vi "VI_Heat_Tape_Final_single_unit.vi"() -> ()   [LabVIEW 2019]
uses:
  <vilib>/NI/Modbus Library/API/Wrapper/Create Serial Master.vi
  <vilib>/NI/Modbus Library/API/Master/Modbus Master.lvclass
  <vilib>/NI/Modbus Library/API/Wrapper/API Main.lvlib
panel:
  out "Value 4":sgl
  out "Connection Status":bool
  in  "unit ID (Defaut: 1)":u8=1
  in  "number of inputs (Defaut: 60)":u16
  in  "starting address (Default: 1)":u16
  in  "Flow Control (Default: None)":u16(ring) items=["None", "XON/XOFF", "RTS/CTS", "XON/XOFF & RTS/CTS", "DTR/DSR", "XON/XOFF & DTR/DSR"]
  in  "Serial Type (Default: RTU)":enum16{"RTU", "ASCII"}(ring)
  in  "Parity (Default: None)":u16(ring)=2 items=["None", "Odd", "Even", "Mark", "Space"]
  in  "Baud Rate (Default: 115400)":u32=9600
  in  "COM Port (Default: COM7)":refnum<visa-resource-name>
  in  "Set Value":string
  out "?":cluster{dbl, dbl}(graph)
  in  "Hysterisis Value":string
  in  "?":bool
  out "Current Temperature (ºF)":string
  in  "error check":errorcluster
  # "SpinQuest Heat Tape Temperature Monitoring System"
  # "PXF4 Settings"
  # "RS-485 Connection"
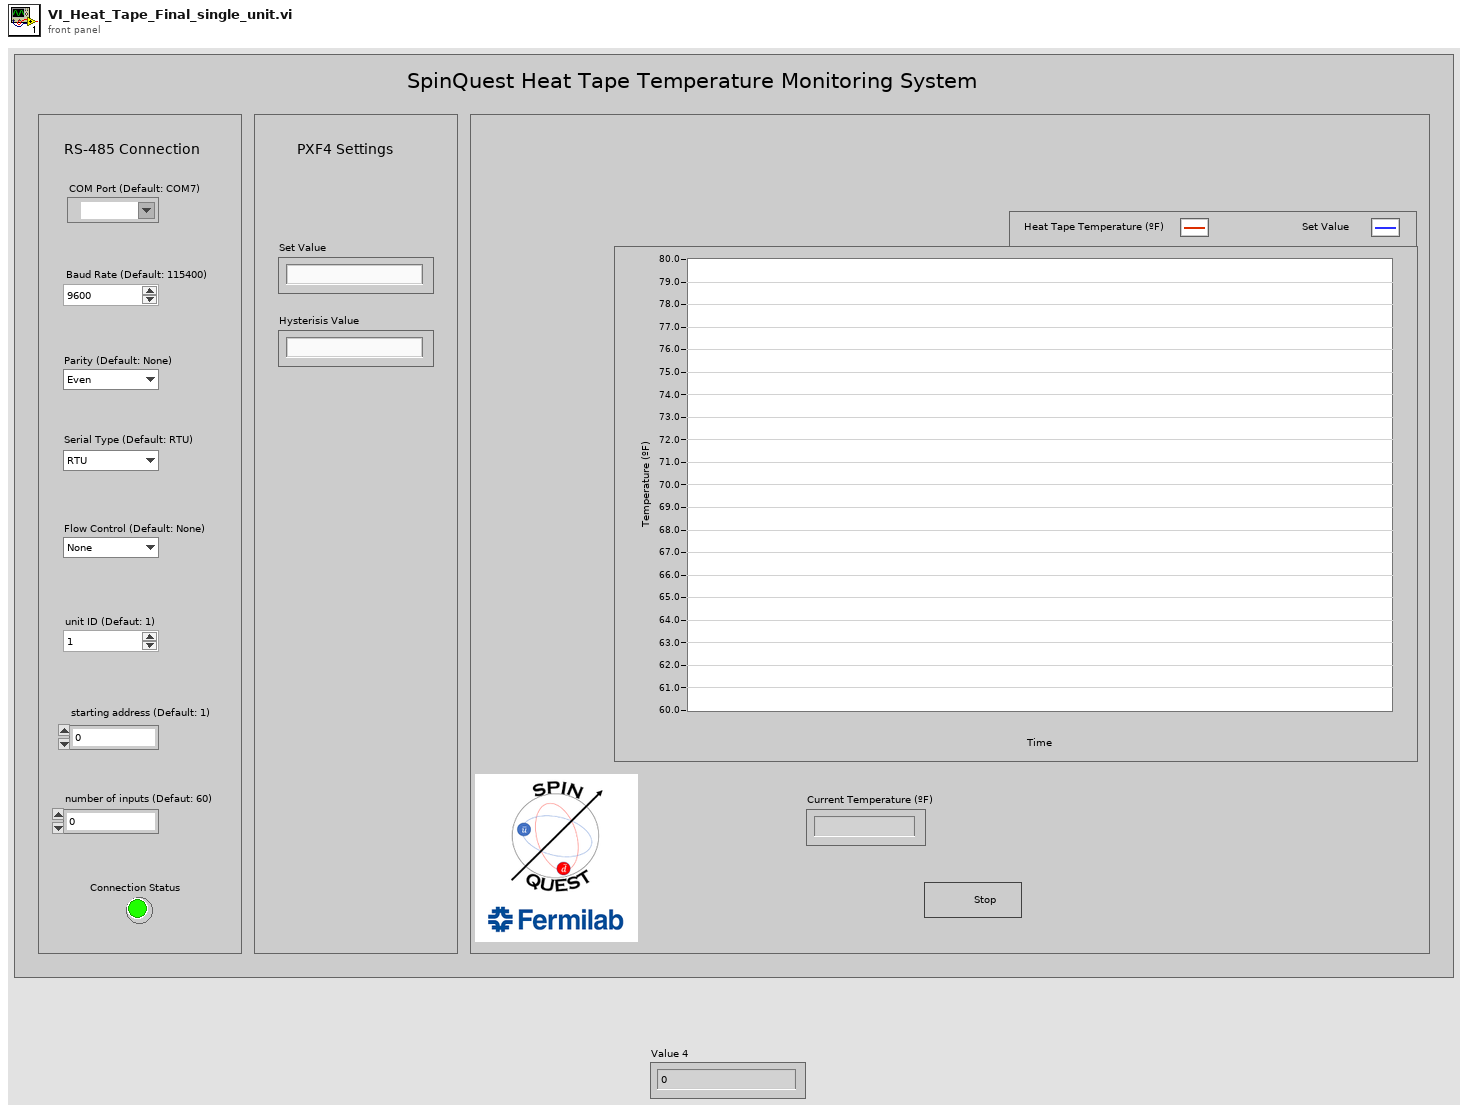
[diagram p1: front panel]
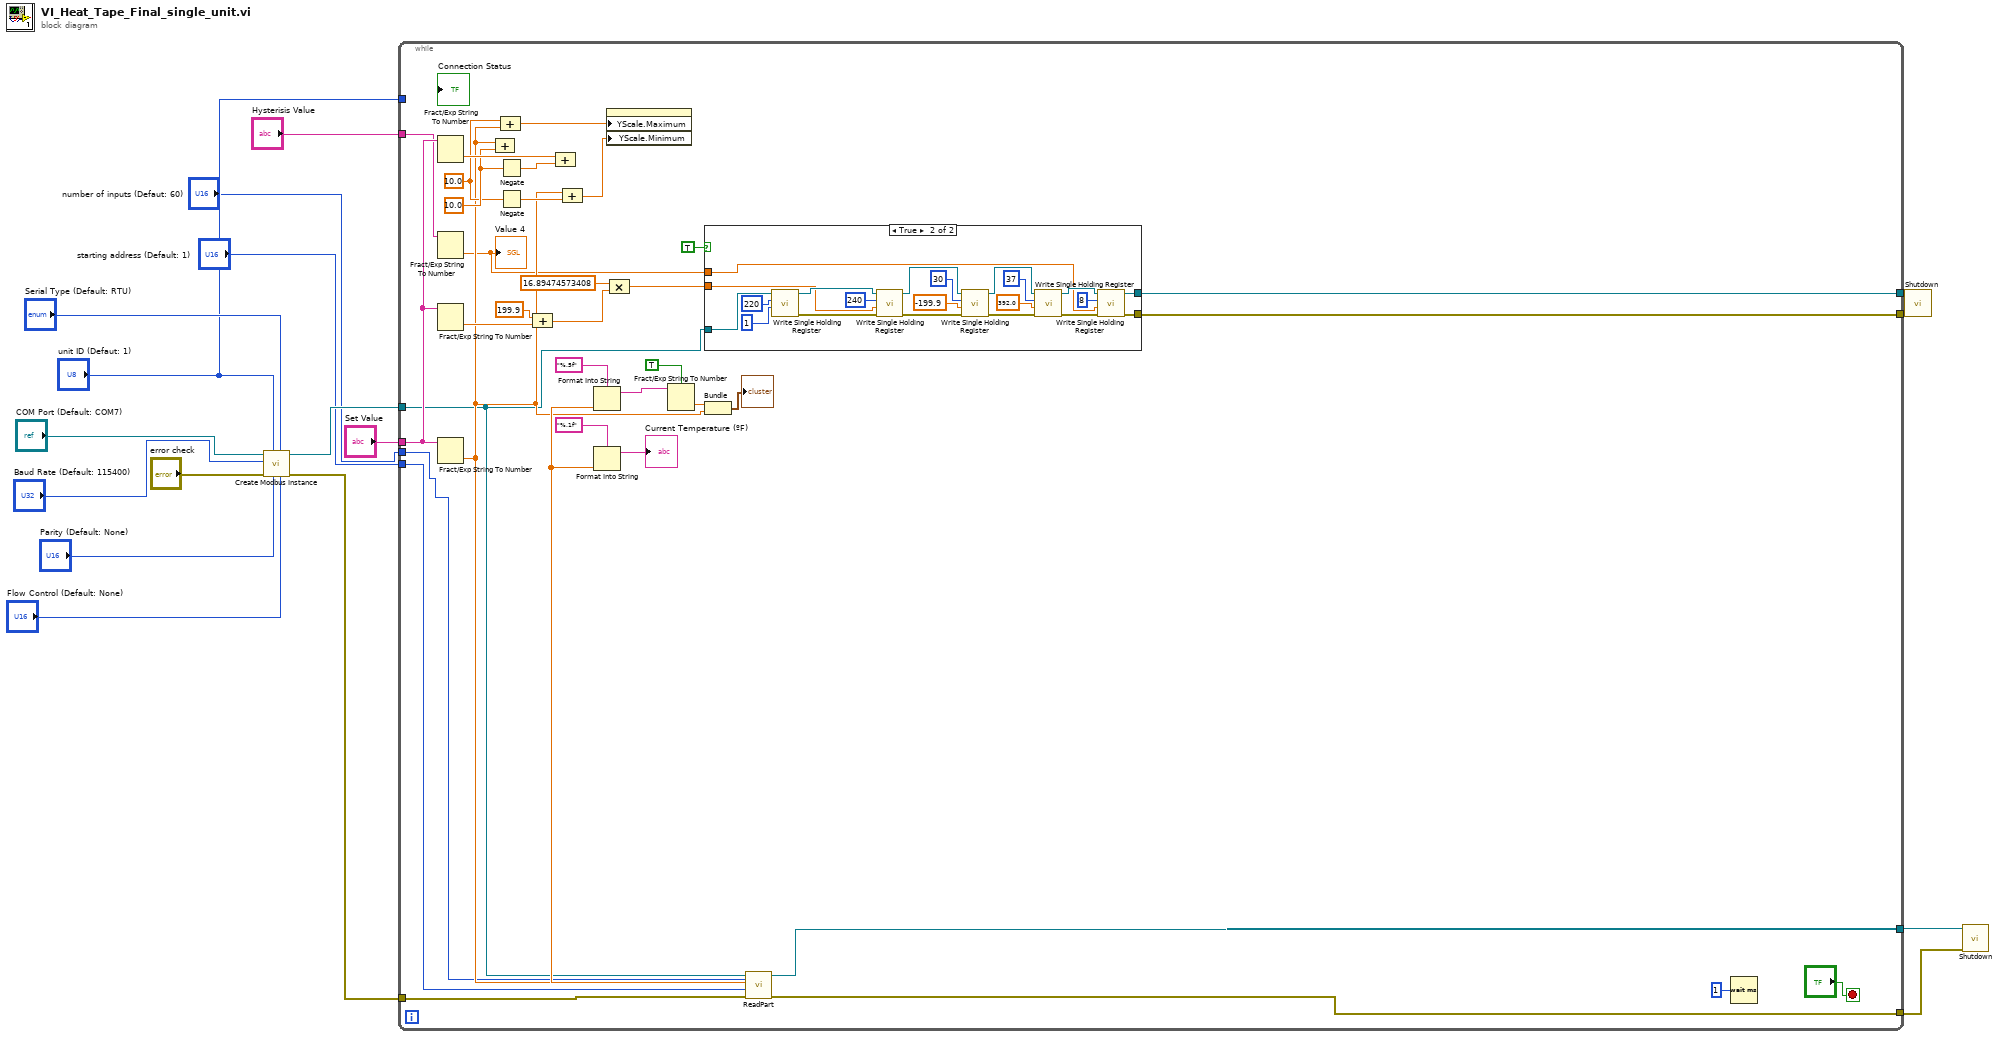
[diagram p0: block diagram]
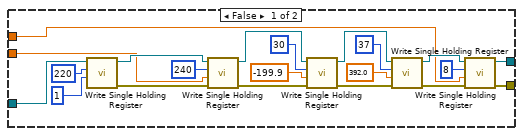
[diagram p2: hidden frame]
diagram:
  n1 = call-poly <vilib>:"Create Modbus Instance.vi"("flow control (none)"="Flow Control (Default: None)", "serial type"="Serial Type (Default: RTU)", "parity (even)"="Parity (Default: None)", "unit ID"="unit ID (Defaut: 1)", "error in"="error check", "baud rate"="Baud Rate (Default: 115400)", "VISA resource name"="COM Port (Default: COM7)") -> ("error out"=w11:errorcluster, "serial master instance"=w12:refnum<class "Modbus Master.lvclass">)  [unwired: 3 in]
  n2 = while {
    tunnel: w12 -> [w20]
    tunnel: w11 -> [w18]
    tunnel: [w45] -> w9
    tunnel: [w39] -> w7
    tunnel: "unit ID (Defaut: 1)" -> [_]
    tunnel: [w24] -> w6
    tunnel: [w25] -> w5
    tunnel: "starting address (Default: 1)" -> [w28]
    tunnel: "number of inputs (Defaut: 60)" -> [w27]
    tunnel: "Set Value" -> [w26]
    tunnel: "Hysterisis Value" -> [w22]
    stop <- "?" stop-if-true
    w34 = 10.0 ("value")
    w41 = 10.0 ("value")
    n3 = Fract/Exp String To Number(string=w26) -> (number=w42:dbl)  [unwired: 3 in, 1 out]
    n4 = Fract/Exp String To Number(string=w22) -> (number=w23:dbl)  [unwired: 3 in, 1 out]
    "Value 4" <- w23
    n5 = Fract/Exp String To Number(string=w26) -> (number=w38:dbl)  [unwired: 3 in, 1 out]
    n6 = Fract/Exp String To Number(string=w26) -> (number=w29:dbl)  [unwired: 3 in, 1 out]
    n7 = Compound Arithmetic op=unknown(w29, w41) -> ()  [unwired: 1 out]
    n8 = Negate(x=w41) -> (-x=w40:dbl)
    n9 = Negate(x=w34) -> (-x=w33:dbl)
    n10 = Compound Arithmetic op=unknown(w34, w29) -> (w32:dbl)
    n11 = Compound Arithmetic op=unknown(199.9 ("value"), w38) -> (w36:dbl)
    n12 = Compound Arithmetic op=unknown(w42, w40) -> ()  [unwired: 1 out]
    n13 = Compound Arithmetic op=unknown(w29, w33) -> (w31:dbl)
    n14 = property class="WFChart (strict)"("YScale.Maximum"=w32, "YScale.Minimum"=w31) -> ()  [unwired: 2 in, 2 out]
    n15 = Compound Arithmetic op=MULTIPLY(16.89474573408 ("value"), w36) -> (w19:dbl)
    n16 = case shown="True" TRUE {
      tunnel: [w61 w84] -> w25
      tunnel: [w60 w82] -> w24
      tunnel: w23 -> [w59 w80]
      tunnel: w20 -> [w56 w77]
      tunnel: w19 -> [w53 w74]
      frame False {
        n17 = call-dynamic "Write Single Holding Register.vi"("register to write"=u16 1, "address"=u16 220, "Modbus master in"=w56) -> ("error out"=w54:errorcluster, "Modbus master out"=w55:refnum<class "Modbus Master.lvclass">)  [unwired: 7 in]
        n18 = call-dynamic "Write Single Holding Register.vi"("error in"=w54, "register to write"=w53, "address"=u16 240, "Modbus master in"=w55) -> ("error out"=w71:errorcluster, "Modbus master out"=w70:refnum<class "Modbus Master.lvclass">)  [unwired: 6 in]
        n19 = call-dynamic "Write Single Holding Register.vi"("error in"=w71, "register to write"=-199.9 ("value"), "address"=u16 30, "Modbus master in"=w70) -> ("error out"=w72:errorcluster, "Modbus master out"=w73:refnum<class "Modbus Master.lvclass">)  [unwired: 6 in]
        n20 = call-dynamic "Write Single Holding Register.vi"("error in"=w72, "register to write"=392.0 ("value"), "address"=u16 37, "Modbus master in"=w73) -> ("error out"=w64:errorcluster, "Modbus master out"=w63:refnum<class "Modbus Master.lvclass">)  [unwired: 6 in]
        n21 = call-dynamic "Write Single Holding Register.vi"("error in"=w64, "register to write"=w59, "address"=u16 8, "Modbus master in"=w63) -> ("error out"=w61:errorcluster, "Modbus master out"=w60:refnum<class "Modbus Master.lvclass">)  [unwired: 6 in]
      }
      frame True {
        n22 = call-dynamic "Write Single Holding Register.vi"("register to write"=u16 1, "address"=u16 220, "Modbus master in"=w77) -> ("error out"=w75:errorcluster, "Modbus master out"=w76:refnum<class "Modbus Master.lvclass">)  [unwired: 7 in]
        n23 = call-dynamic "Write Single Holding Register.vi"("error in"=w75, "register to write"=w74, "address"=u16 240, "Modbus master in"=w76) -> ("error out"=w92:errorcluster, "Modbus master out"=w91:refnum<class "Modbus Master.lvclass">)  [unwired: 6 in]
        n24 = call-dynamic "Write Single Holding Register.vi"("error in"=w92, "register to write"=-199.9 ("value"), "address"=u16 30, "Modbus master in"=w91) -> ("error out"=w93:errorcluster, "Modbus master out"=w94:refnum<class "Modbus Master.lvclass">)  [unwired: 6 in]
        n25 = call-dynamic "Write Single Holding Register.vi"("error in"=w93, "register to write"=392.0 ("value"), "address"=u16 37, "Modbus master in"=w94) -> ("error out"=w85:errorcluster, "Modbus master out"=w83:refnum<class "Modbus Master.lvclass">)  [unwired: 6 in]
        n26 = call-dynamic "Write Single Holding Register.vi"("error in"=w85, "register to write"=w80, "address"=u16 8, "Modbus master in"=w83) -> ("error out"=w84:errorcluster, "Modbus master out"=w82:refnum<class "Modbus Master.lvclass">)  [unwired: 6 in]
      }
    }
    n27 = call "ReadPart.vi"("number of inputs (Defaut: 60)"=w27, "error in (no error)"=w18, "starting address (Default: 1)"=w28, "Numeric in"=w29, "Modbus Master in"=w20) -> ("error out"=w45:errorcluster, "Numeric out"=w30:dbl, "Modbus Master out"=w39:refnum<class "Modbus Master.lvclass">)  [unwired: 4 in]
    n28 = Format Into String(format string="%.5f", w30) -> (resulting string=w47:string)  [unwired: 2 in, 1 out]
    n29 = Format Into String(format string="%.1f", w30) -> (resulting string=→"Current Temperature (ºF)":string)  [unwired: 2 in, 1 out]
    n30 = Fract/Exp String To Number(use system decimal point (T)=TRUE, string=w47) -> (number=w44:dbl)  [unwired: 2 in, 1 out]
    n31 = Bundle(w44, w29) -> (→"?":cluster{dbl, dbl})  [unwired: 1 in]
    n32 = Wait (ms)(milliseconds to wait=u32 1) -> ()  [unwired: 1 out]
  }
  n33 = call-dynamic "Shutdown.vi"("error in"=w5, "Modbus master in"=w6) -> ()  [unwired: 9 in, 1 out]
  n34 = call-dynamic "Shutdown.vi"("error in"=w9, "Modbus master in"=w7) -> ()  [unwired: 9 in, 1 out]
